vi "ReadDataUseNotifier.vi"(8 "error in (no error)":errorcluster, 11 "notifierIn":refnum<notifier>) -> (0 "error out":errorcluster, 2 "Data":T1, 3 "notifier out":refnum<notifier>)   [LabVIEW 2012, in "DataBank.lvclass"]
uses:
  DataBank.lvclass
  DataBank.lvclass/DataBank.ctl
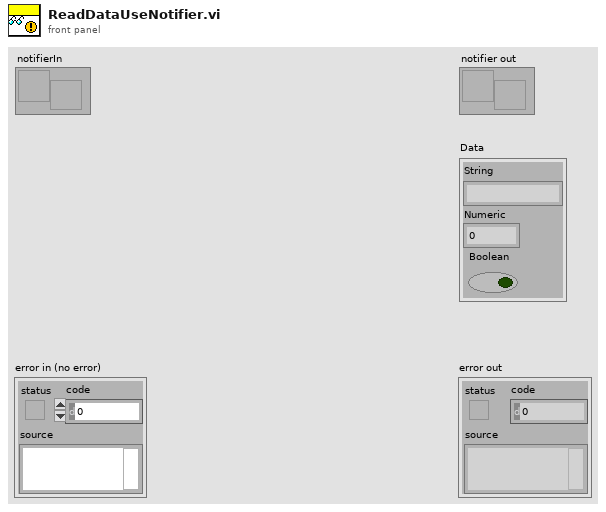
[diagram p1: front panel]
types:
  T1 = cluster{"String":string, "Numeric":i32, "Boolean":bool}
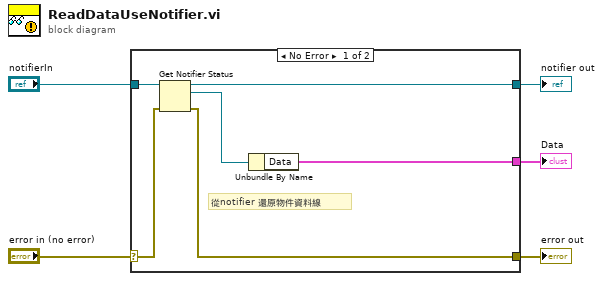
[diagram p0: block diagram]
diagram:
  n1 = case shown="No Error" "error in (no error)" {
    selector: "error in (no error)" -> [w7 w12]
    tunnel: [w6 w12] -> w4
    tunnel: [w9 w13] -> w2
    tunnel: "notifierIn" -> [w10 w13]
    tunnel: [w11 _] -> w1
    frame No Error {
      # "從notifier 還原物件資料線"
      n2 = Get Notifier Status(notifier=w10, error in (no error)=w7) -> (notifier out=w9:refnum<notifier>, current notification=w8:refnum<class "DataBank.lvclass">, error out=w6:errorcluster)  [unwired: 2 out]
      n3 = Unbundle By Name(w8) -> ("Data"=w11:T1)
    }
    frame Error {
    }
  }
  "error out" <- w4
  "notifier out" <- w2
  "Data" <- w1
